vi "6733_write_waveform_2014.11.21.vi"(8 "Error In":errorcluster, 9 "Control Reference \nCluster Input":T1, 11 "Red MOT 87 Inputs 2":T2={"Active Device"="6733_Red_87", "Active Channels"=[TRUE, TRUE, TRUE, TRUE, FALSE, FALSE, FALSE, FALSE], "Waveform Parameters"=[[{"Function"=enum."Exponential", "Initial"=0.0, "Final"=0.0, "Degree"=1.0, "Nickname"="", "Conversion"=enum."B Field Grad (G/cm)", "Constant"=0.0}, {"Function"=enum."Exponential", "Initial"=0.0, "Final"=0.0, "Degree"=1.0, "Nickname"="", "Conversion"=enum."B Field Grad (G/cm)", "Constant"=0.0}, {"Function"=enum."Exponential", "Initial"=0.0, "Final"=0.0, "Degree"=1.0, "Nickname"="", "Conversion"=enum."B Field Grad (G/cm)", "Constant"=0.0}, {"Function"=enum."Exponential", "Initial"=0.0, "Final"=0.0, "Degree"=1.0, "Nickname"="", "Conversion"=enum."B Field Grad (G/cm)", "Constant"=0.0}, {"Function"=enum."Exponential", "Initial"=0.0, "Final"=0.0, "Degree"=1.0, "Nickname"="", "Conversion"=enum."B Field Grad (G/cm)", "Constant"=0.0}, {"Function"=enum."Exponential", "Initial"=0.0, "Final"=0.0, "Degree"=1.0, "Nickname"="", "Conversion"=enum."B Field Grad (G/cm)", "Constant"=0.0}], [{"Function"=enum."Exponential", "Initial"=0.0, "Final"=0.0, "Degree"=1.0, "Nickname"="", "Conversion"=enum."B Field Grad (G/cm)", "Constant"=0.0}, {"Function"=enum."Exponential", "Initial"=0.0, "Final"=0.0, "Degree"=1.0, "Nickname"="", "Conversion"=enum."B Field Grad (G/cm)", "Constant"=0.0}, {"Function"=enum."Exponential", "Initial"=0.0, "Final"=0.0, "Degree"=1.0, "Nickname"="", "Conversion"=enum."B Field Grad (G/cm)", "Constant"=0.0}, {"Function"=enum."Exponential", "Initial"=0.0, "Final"=0.0, "Degree"=1.0, "Nickname"="", "Conversion"=enum."B Field Grad (G/cm)", "Constant"=0.0}, {"Function"=enum."Exponential", "Initial"=0.0, "Final"=0.0, "Degree"=1.0, "Nickname"="", "Conversion"=enum."B Field Grad (G/cm)", "Constant"=0.0}, {"Function"=enum."Exponential", "Initial"=0.0, "Final"=0.0, "Degree"=1.0, "Nickname"="", "Conversion"=enum."B Field Grad (G/cm)", "Constant"=0.0}], [{"Function"=enum."Exponential", "Initial"=0.0, "Final"=0.0, "Degree"=1.0, "Nickname"="", "Conversion"=enum."B Field Grad (G/cm)", "Constant"=0.0}, {"Function"=enum."Exponential", "Initial"=0.0, "Final"=0.0, "Degree"=1.0, "Nickname"="", "Conversion"=enum."B Field Grad (G/cm)", "Constant"=0.0}, {"Function"=enum."Exponential", "Initial"=0.0, "Final"=0.0, "Degree"=1.0, "Nickname"="", "Conversion"=enum."B Field Grad (G/cm)", "Constant"=0.0}, {"Function"=enum."Exponential", "Initial"=0.0, "Final"=0.0, "Degree"=1.0, "Nickname"="", "Conversion"=enum."B Field Grad (G/cm)", "Constant"=0.0}, {"Function"=enum."Exponential", "Initial"=0.0, "Final"=0.0, "Degree"=1.0, "Nickname"="", "Conversion"=enum."B Field Grad (G/cm)", "Constant"=0.0}, {"Function"=enum."Exponential", "Initial"=0.0, "Final"=0.0, "Degree"=1.0, "Nickname"="", "Conversion"=enum."B Field Grad (G/cm)", "Constant"=0.0}], [{"Function"=enum."Exponential", "Initial"=0.0, "Final"=0.0, "Degree"=1.0, "Nickname"="", "Conversion"=enum."B Field Grad (G/cm)", "Constant"=0.0}, {"Function"=enum."Exponential", "Initial"=0.0, "Final"=0.0, "Degree"=1.0, "Nickname"="", "Conversion"=enum."B Field Grad (G/cm)", "Constant"=0.0}, {"Function"=enum."Exponential", "Initial"=0.0, "Final"=0.0, "Degree"=1.0, "Nickname"="", "Conversion"=enum."B Field Grad (G/cm)", "Constant"=0.0}, {"Function"=enum."Exponential", "Initial"=0.0, "Final"=0.0, "Degree"=1.0, "Nickname"="", "Conversion"=enum."B Field Grad (G/cm)", "Constant"=0.0}, {"Function"=enum."Exponential", "Initial"=0.0, "Final"=0.0, "Degree"=1.0, "Nickname"="", "Conversion"=enum."B Field Grad (G/cm)", "Constant"=0.0}, {"Function"=enum."Exponential", "Initial"=0.0, "Final"=0.0, "Degree"=1.0, "Nickname"="", "Conversion"=enum."B Field Grad (G/cm)", "Constant"=0.0}], [{"Function"=enum."Exponential", "Initial"=0.0, "Final"=0.0, "Degree"=1.0, "Nickname"="", "Conversion"=enum."B Field Grad (G/cm)", "Constant"=0.0}, {"Function"=enum."Exponential", "Initial"=0.0, "Final"=0.0, "Degree"=1.0, "Nickname"="", "Conversion"=enum."B Field Grad (G/cm)", "Constant"=0.0}, {"Function"=enum."Exponential", "Initial"=0.0, "Final"=0.0, "Degree"=1.0, "Nickname"="", "Conversion"=enum."B Field Grad (G/cm)", "Constant"=0.0}, {"Function"=enum."Exponential", "Initial"=0.0, "Final"=0.0, "Degree"=1.0, "Nickname"="", "Conversion"=enum."B Field Grad (G/cm)", "Constant"=0.0}, {"Function"=enum."Exponential", "Initial"=0.0, "Final"=0.0, "Degree"=1.0, "Nickname"="", "Conversion"=enum."B Field Grad (G/cm)", "Constant"=0.0}, {"Function"=enum."Exponential", "Initial"=0.0, "Final"=0.0, "Degree"=1.0, "Nickname"="", "Conversion"=enum."B Field Grad (G/cm)", "Constant"=0.0}], [{"Function"=enum."Exponential", "Initial"=0.0, "Final"=0.0, "Degree"=1.0, "Nickname"="", "Conversion"=enum."B Field Grad (G/cm)", "Constant"=0.0}, {"Function"=enum."Exponential", "Initial"=0.0, "Final"=0.0, "Degree"=1.0, "Nickname"="", "Conversion"=enum."B Field Grad (G/cm)", "Constant"=0.0}, {"Function"=enum."Exponential", "Initial"=0.0, "Final"=0.0, "Degree"=1.0, "Nickname"="", "Conversion"=enum."B Field Grad (G/cm)", "Constant"=0.0}, {"Function"=enum."Exponential", "Initial"=0.0, "Final"=0.0, "Degree"=1.0, "Nickname"="", "Conversion"=enum."B Field Grad (G/cm)", "Constant"=0.0}, {"Function"=enum."Exponential", "Initial"=0.0, "Final"=0.0, "Degree"=1.0, "Nickname"="", "Conversion"=enum."B Field Grad (G/cm)", "Constant"=0.0}, {"Function"=enum."Exponential", "Initial"=0.0, "Final"=0.0, "Degree"=1.0, "Nickname"="", "Conversion"=enum."B Field Grad (G/cm)", "Constant"=0.0}], [{"Function"=enum."Exponential", "Initial"=0.0, "Final"=0.0, "Degree"=1.0, "Nickname"="", "Conversion"=enum."B Field Grad (G/cm)", "Constant"=0.0}, {"Function"=enum."Exponential", "Initial"=0.0, "Final"=0.0, "Degree"=1.0, "Nickname"="", "Conversion"=enum."B Field Grad (G/cm)", "Constant"=0.0}, {"Function"=enum."Exponential", "Initial"=0.0, "Final"=0.0, "Degree"=1.0, "Nickname"="", "Conversion"=enum."B Field Grad (G/cm)", "Constant"=0.0}, {"Function"=enum."Exponential", "Initial"=0.0, "Final"=0.0, "Degree"=1.0, "Nickname"="", "Conversion"=enum."B Field Grad (G/cm)", "Constant"=0.0}, {"Function"=enum."Exponential", "Initial"=0.0, "Final"=0.0, "Degree"=1.0, "Nickname"="", "Conversion"=enum."B Field Grad (G/cm)", "Constant"=0.0}, {"Function"=enum."Exponential", "Initial"=0.0, "Final"=0.0, "Degree"=1.0, "Nickname"="", "Conversion"=enum."B Field Grad (G/cm)", "Constant"=0.0}], [{"Function"=enum."Exponential", "Initial"=0.0, "Final"=0.0, "Degree"=1.0, "Nickname"="", "Conversion"=enum."B Field Grad (G/cm)", "Constant"=0.0}, {"Function"=enum."Exponential", "Initial"=0.0, "Final"=0.0, "Degree"=1.0, "Nickname"="", "Conversion"=enum."B Field Grad (G/cm)", "Constant"=0.0}, {"Function"=enum."Exponential", "Initial"=0.0, "Final"=0.0, "Degree"=1.0, "Nickname"="", "Conversion"=enum."B Field Grad (G/cm)", "Constant"=0.0}, {"Function"=enum."Exponential", "Initial"=0.0, "Final"=0.0, "Degree"=1.0, "Nickname"="", "Conversion"=enum."B Field Grad (G/cm)", "Constant"=0.0}, {"Function"=enum."Exponential", "Initial"=0.0, "Final"=0.0, "Degree"=1.0, "Nickname"="", "Conversion"=enum."B Field Grad (G/cm)", "Constant"=0.0}, {"Function"=enum."Exponential", "Initial"=0.0, "Final"=0.0, "Degree"=1.0, "Nickname"="", "Conversion"=enum."B Field Grad (G/cm)", "Constant"=0.0}]], "Active Phases"=[TRUE, TRUE, TRUE, FALSE, FALSE, FALSE], "Phase Times"=[0.1, 0.1, 0.1], "Trigger Channel"="/6733_Red_87/PFI0"} {"Phase Times" format="%.0p"; "Waveform Parameters"."Degree" min=1.0}) -> (0 "error out":errorcluster, 2 "counter task out":refnum<k21>, 3 "waveform task out":refnum<k21>)   [LabVIEW 2016]
uses:
  6733_Red_MOT/6733_control_panel.ctl
  6733_Red_MOT/6733_waveform_parameter_array.ctl
  6733_Red_MOT/6733_waveform_item.ctl
  6733_Red_MOT/Neutral_voltage_conversion_control.ctl
  Controls/6733/Trigger_Channel_Selector.ctl
  Control 1.ctl
  <vilib>/DAQmx/write.llb/DAQmx Write (Analog 1D DBL NChan 1Samp).vi
  <vilib>/DAQmx/write.llb/DAQmx Write (Analog 1D Wfm NChan NSamp).vi
  <vilib>/DAQmx/miscellaneous.llb/DAQmx Fill In Error Info.vi
  <vilib>/Waveform/WDTOps.llb/WDT Append Waveforms DBL.vi
  <vilib>/Waveform/WDTOps.llb/WDT Scale Delta t DBL.vi
  <vilib>/DAQmx/configure/timing.llb/DAQmx Timing (Sample Clock).vi
  <vilib>/DAQmx/create/channels.llb/DAQmx Create Channel (CO-Pulse Generation-Frequency).vi
  <vilib>/DAQmx/configure/timing.llb/DAQmx Timing (Implicit).vi
  <vilib>/DAQmx/configure/trigger.llb/DAQmx Start Trigger (Digital Edge).vi
  <resource>/objmgr/daqmx.rc
panel:
  out "Total Time":dbl
  out "Sample Rate":dbl
  out "Waveforms":waveform(dbl)[](array[waveform])
  out "Max Sample Rate":dbl=1000000.0
  out "Num Inactive":i32
  out "Num  Active":i32
  out "Inactive Channels":tag[](array[tag])
  out "Active Channels":tag[](array[tag])
  out "Samples Written":dbl
  out "Voltage Maximum":dbl
  out "Voltage Minimum":dbl
  out "AO.PhysicalChans":tag[](array[tag])
  out "Active Device":tag
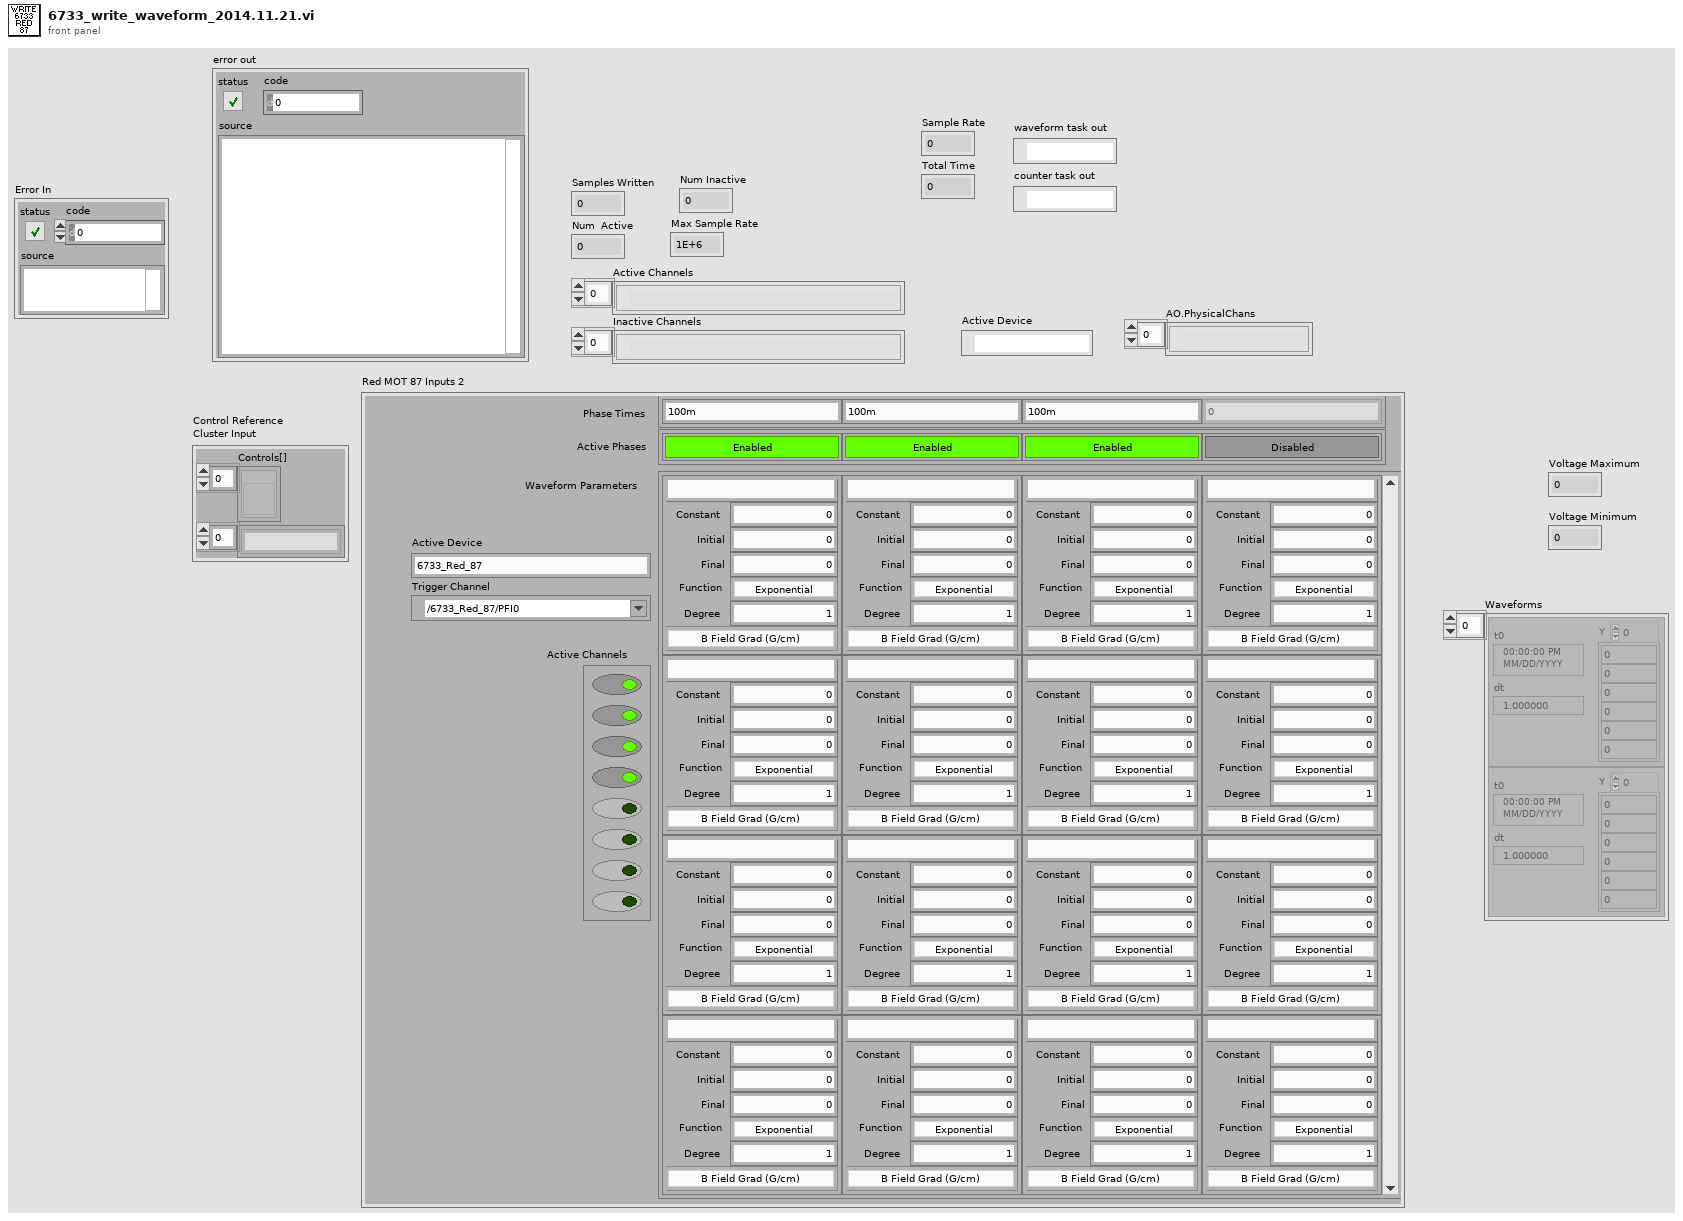
[diagram p1: front panel]
types:
  T1 = cluster{"Controls[]":refnum<vi>[], "Control Names":string[]}
  T2 = typedef "6733_control_panel.ctl" = cluster{"Active Device":string, "Active Channels":bool[], "Waveform Parameters":T3, "Active Phases":bool[], "Phase Times":dbl[], "Trigger Channel":T6}
  T3 = typedef "6733_waveform_parameter_array.ctl" = T4[][]
  T4 = typedef "6733_waveform_item.ctl" = cluster{"Function":enum16{"Polynomial", "Exponential", "Constant", "Tanh"}, "Initial":dbl, "Final":dbl, "Degree":dbl, "Nickname":string, "Conversion":T5, "Constant":dbl}
  T5 = typedef "Neutral_voltage_conversion_control.ctl" = enum16{"Volts", "B Field Grad (G/cm)", "Red Boson Cntr Freq (MHz)", "Red Boson Dither Amp (kHz)", "Red Boson Power (mW)", "Red 87 Trap Cntr Freq (MHz)", "Red 87 Trap Dither Amp (kHz)", "Red 87 Trap Power (mW)", "Red 87 Stir Cntr Freq (MHz)", "Red 87 Stir Dither Amp (kHz)", "Red 87 Stir Power (mW)", "ODT Sheet Trap Power (W)", "ODT Loading Trap Power (W)"}
  T6 = typedef "Trigger_Channel_Selector.ctl" = tag
  T7 = typedef "Control 1.ctl" = enum16{"Initialize", "Get Device Information", "Get Active/Inactive Channels", "Maximize Samples / Channel", "Calculate Waveforms", "Check for Problems", "Update Front Panel", "Clear Old Tasks", "Write Initialization to Cards", "Write Waveform to Cards"}
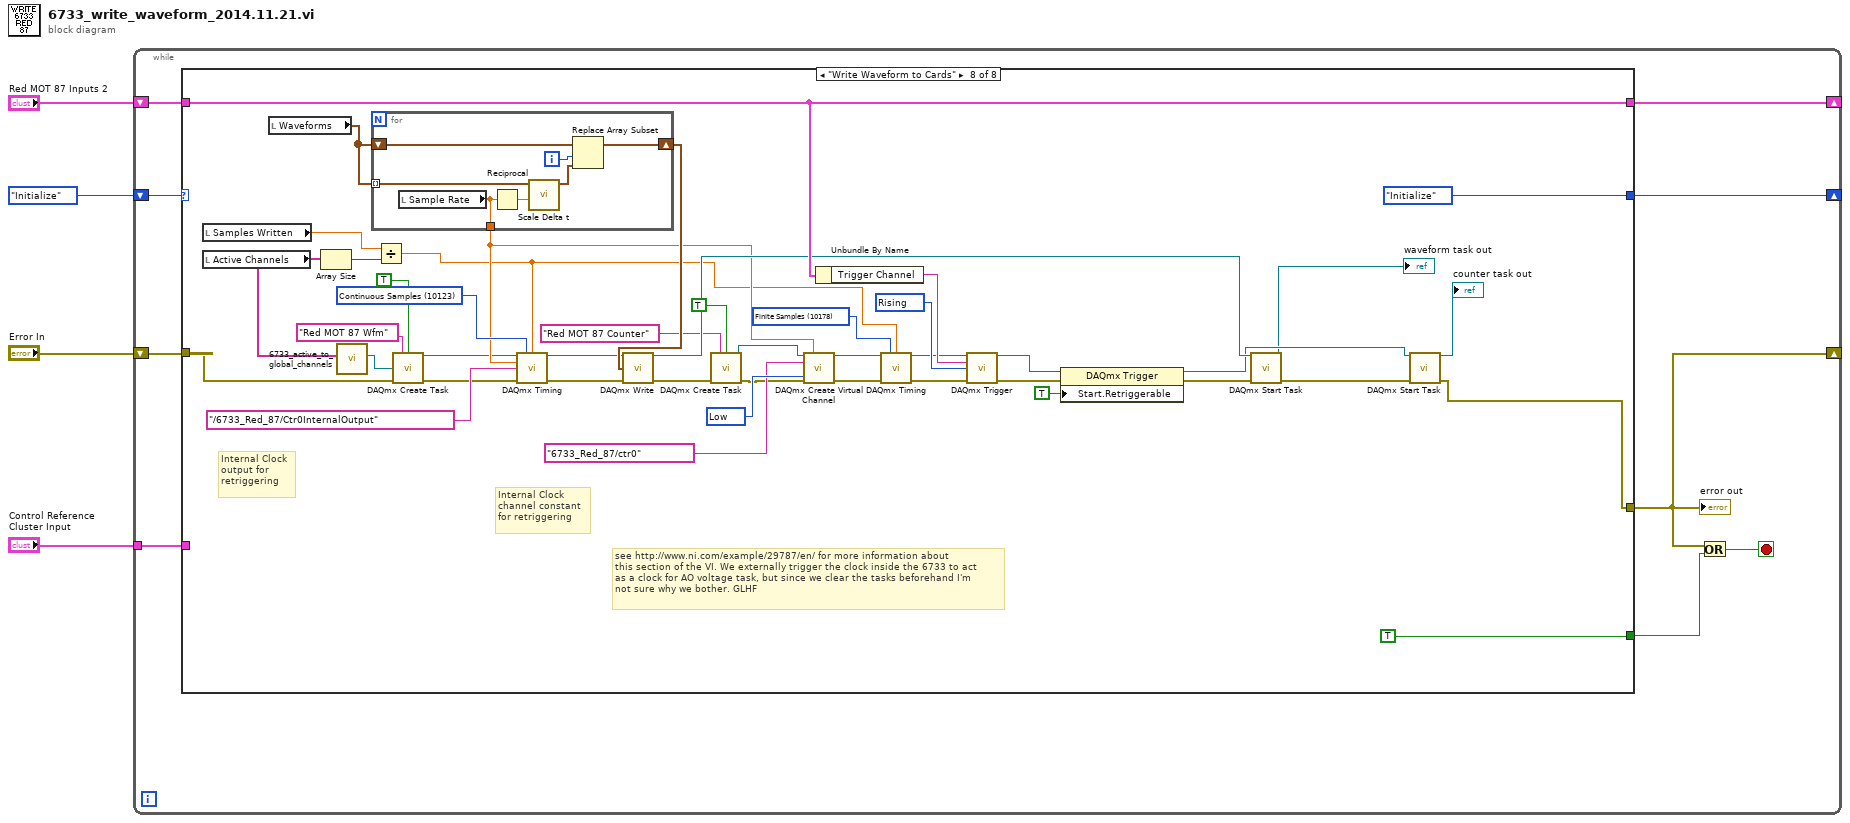
[diagram p0: block diagram]
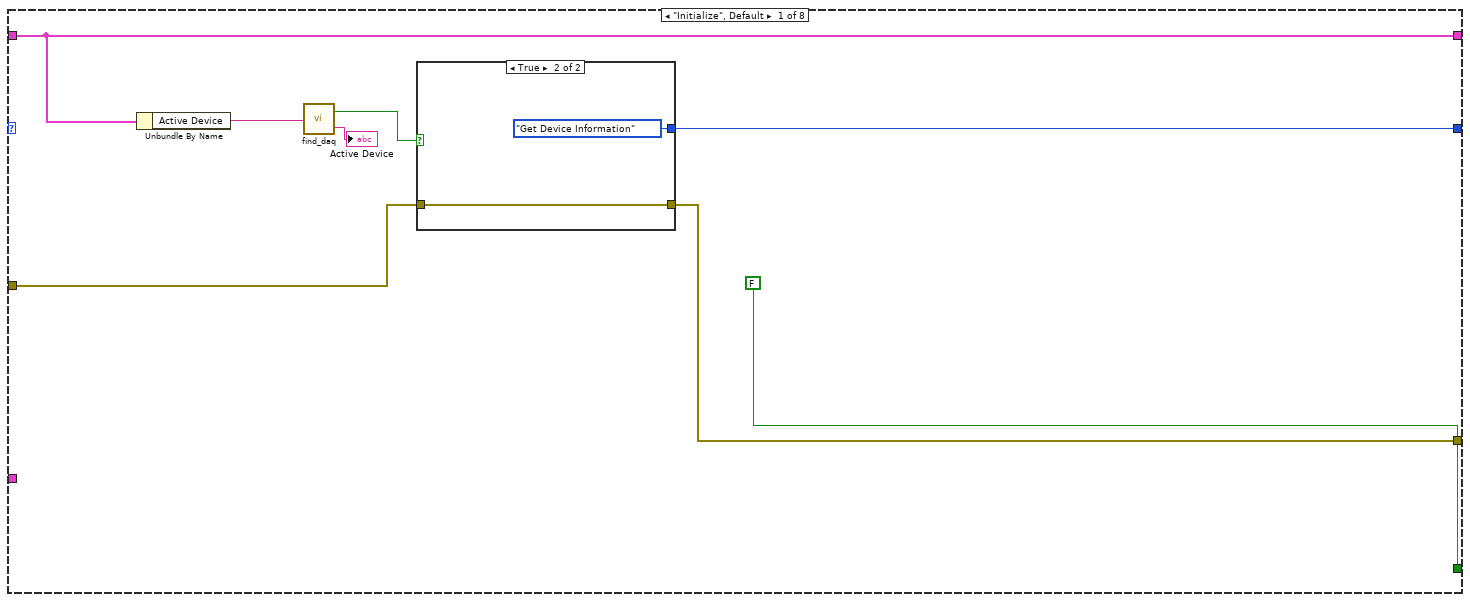
[diagram p2: hidden frame]
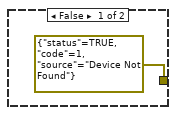
[diagram p3: hidden frame]
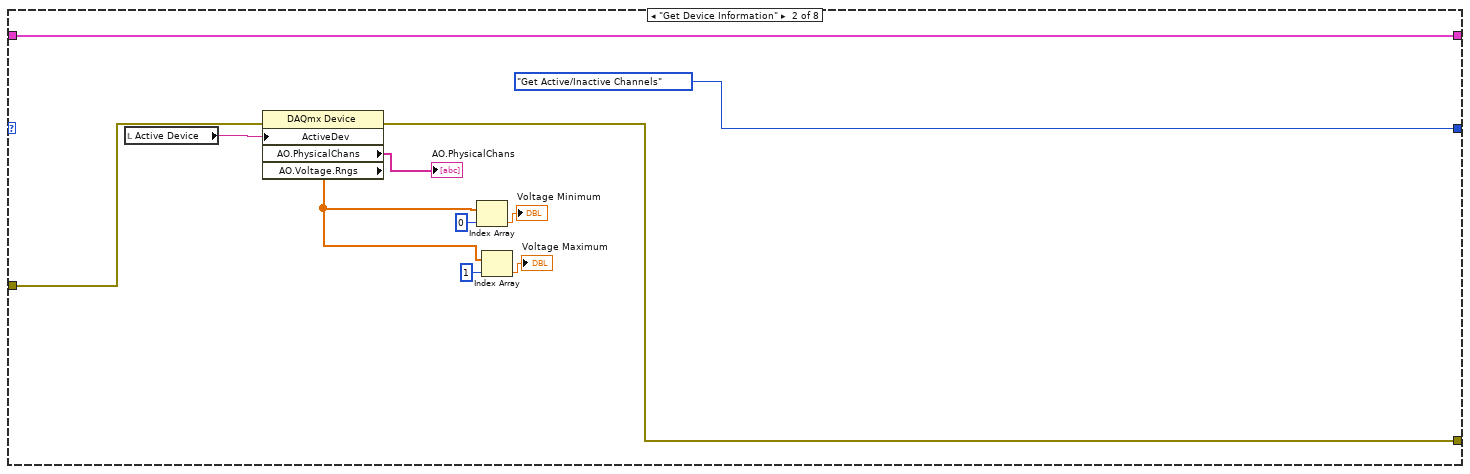
[diagram p4: hidden frame]
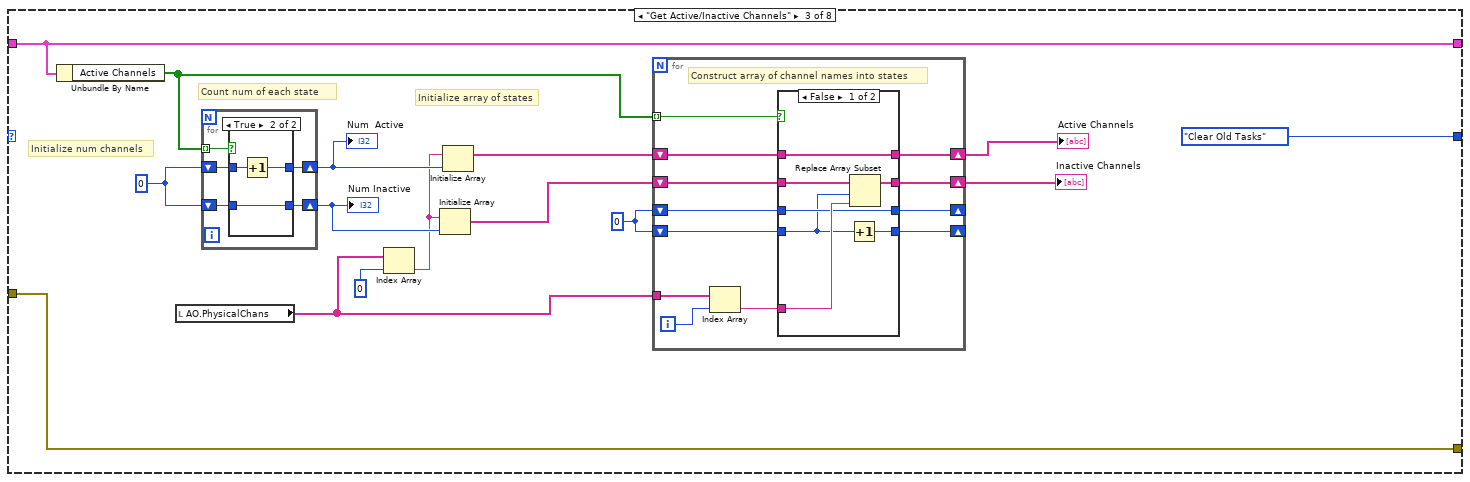
[diagram p5: hidden frame]
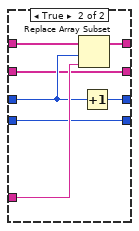
[diagram p6: hidden frame]
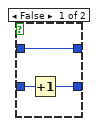
[diagram p7: hidden frame]
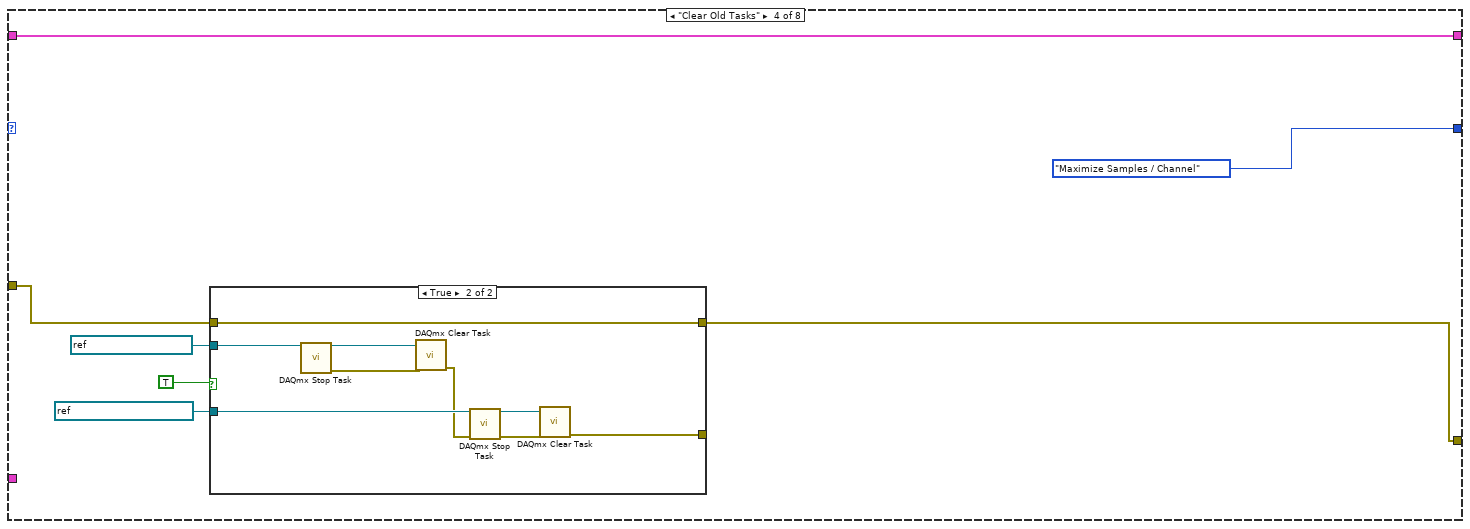
[diagram p8: hidden frame]
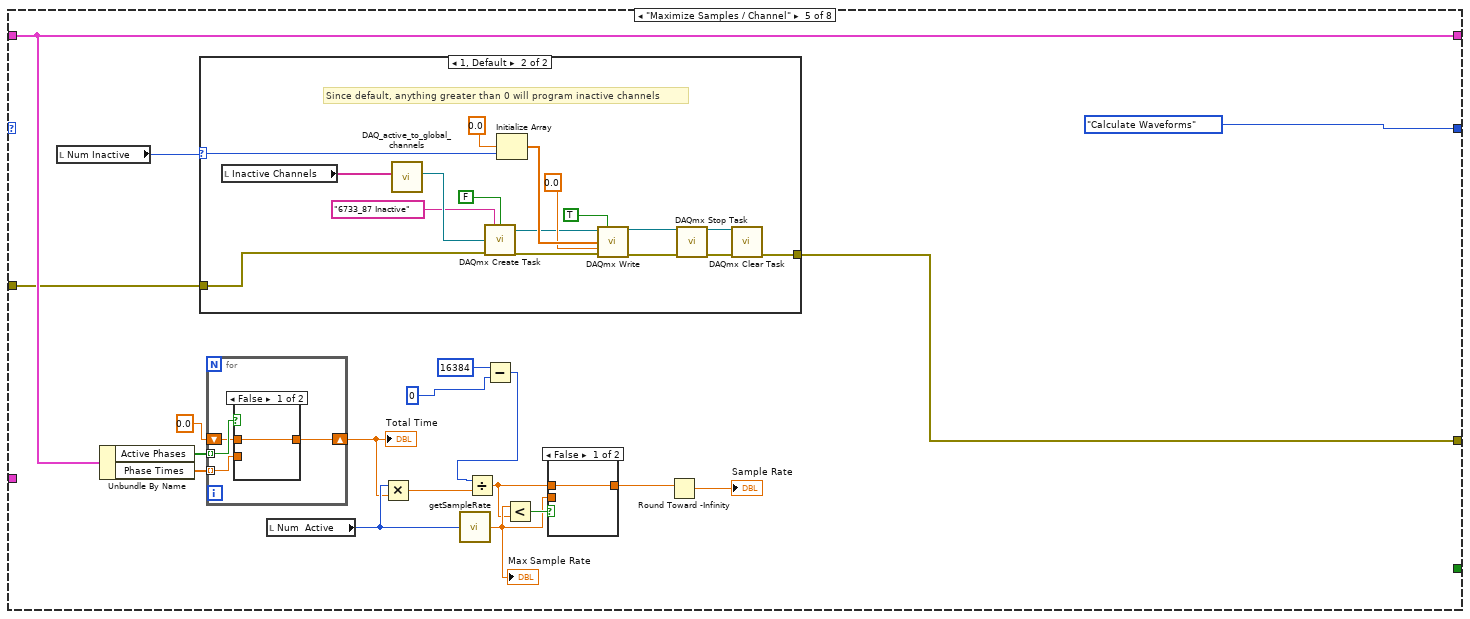
[diagram p10: hidden frame]
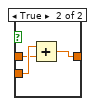
[diagram p13: hidden frame]
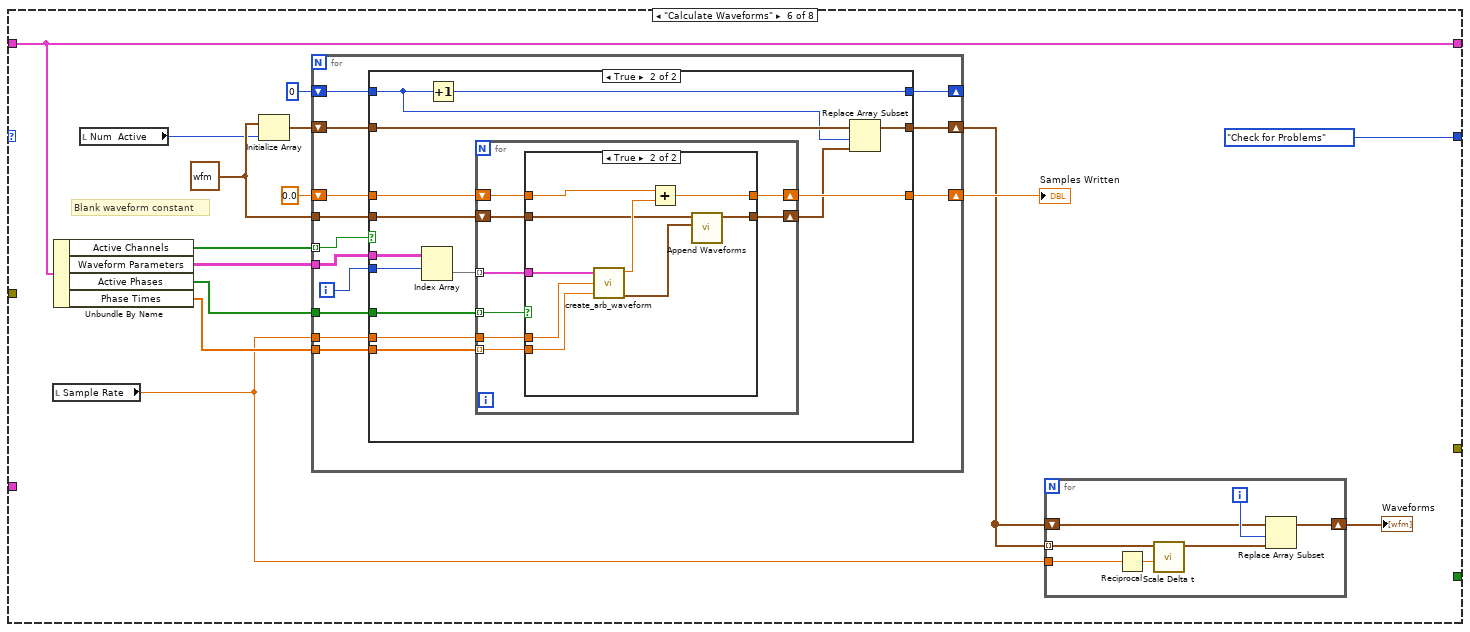
[diagram p14: hidden frame]
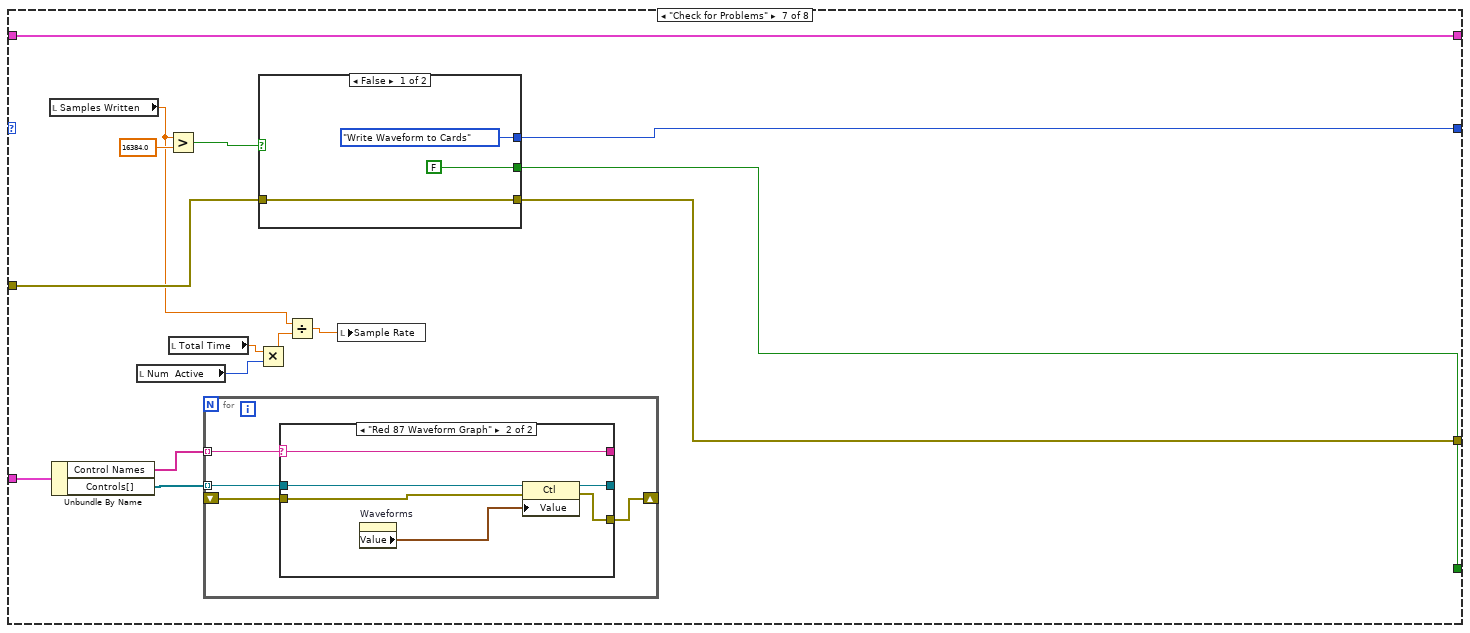
[diagram p17: hidden frame]
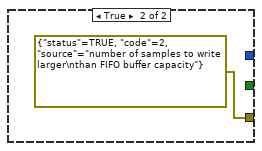
[diagram p19: hidden frame]
diagram:
  n1 = while {
    shift-right: [w5] -> _
    shift-left: "Error In" -> [w11]
    shift-right: [w10] -> _
    shift-left: Control_1."Initialize" -> [w13]
    shift-right: [w8] -> _
    shift-left: "Red MOT 87 Inputs 2" -> [w12]
    tunnel: "Control Reference \nCluster Input" -> [w6]
    stop <- w9 stop-if-true
    n2 = case shown="\"Write Waveform to Cards\"" w13 {
      tunnel: w12 -> [w15 w35 w41 w90 w121 w163 w233 w296]
      tunnel: [w18 w26 w50 w93 w123 _ w234 w273] -> w5
      tunnel: w11 -> [w17 w34 w50 w92 w106 _ w235 w270]
      tunnel: [w16 Control_1."Get Active/Inactive Channels" Control_1."Clear Old Tasks" Control_1."Maximize Samples / Channel" Control_1."Calculate Waveforms" Control_1."Check for Problems" w232 Control_1."Initialize"] -> w10
      tunnel: [w15 w35 w41 w90 w121 w163 w233 w296] -> w8
      tunnel: [FALSE ("y") _ _ _ _ _ w231 TRUE ("y")] -> w7
      tunnel: w6 -> [_ _ _ _ _ _ w223 _]
      frame "Initialize", Default {
        n3 = Unbundle By Name(w15) -> ("Active Device"=w21:string)
        n4 = call "find_daq.vi"("Device Name"=w21) -> ("Device Present"=w19:bool, "DAQmx Device Name"=→"Active Device":tag)
        n5 = case shown="True" w19 {
          tunnel: [errorcluster {"status"=TRUE, "code"=1, "source"="Device Not Found"} ("error in (no error)") w24] -> w18
          tunnel: w17 -> [_ w24]
          tunnel: [_ Control_1."Get Device Information"] -> w16
          frame False {
          }
          frame True {
          }
        }
      }
      frame "Get Device Information" {
        n6 = local read "Active Device"() -> (w33:tag)
        n7 = property class="DAQmx Device"(error in=w34, "ActiveDev"=w33) -> (error out=w26:errorcluster, "AO.PhysicalChans"=→"AO.PhysicalChans":tag[], "AO.Voltage.Rngs"=w28:dbl[])  [unwired: 1 in, 1 out]
        n8 = Index Array(array=w28, index=0) -> (element=→"Voltage Minimum":dbl)
        n9 = Index Array(array=w28, index=1) -> (element=→"Voltage Maximum":dbl)
      }
      frame "Get Active/Inactive Channels" {
        w37 = 0 ("index")
        w36 = 0
        # "Initialize array of states"
        # "Count num of each state"
        # "Initialize num channels"
        n10 = Unbundle By Name(w41) -> ("Active Channels"=w49:bool[])
        n11 = local read "AO.PhysicalChans"() -> (w43:tag[])
        n12 = for {
          shift-right: [w81] -> w48
          shift-left: w36 -> [w80]
          shift-right: [w79] -> w47
          shift-left: w36 -> [w78]
          tunnel: w49 -> [w77] mode=indexing
          n13 = case shown="True" w77 {
            tunnel: [w82 w87] -> w81
            tunnel: w80 -> [w82 w86]
            tunnel: [w84 w85] -> w79
            tunnel: w78 -> [w83 w85]
            frame False {
              n14 = Increment(x=w83) -> (x+1=w84:i32)
            }
            frame True {
              n15 = Increment(x=w86) -> (x+1=w87:i32)
            }
          }
        }
        "Num  Active" <- w48
        "Num Inactive" <- w47
        n16 = Index Array(array=w43, index=0) -> (element=w44:tag)
        n17 = Initialize Array(w44, w47) -> (w42:tag[])
        n18 = Initialize Array(w44, w48) -> (w46:tag[])
        n19 = for {
          tunnel: w49 -> [w62] mode=indexing
          shift-right: [w59] -> w40
          shift-left: w46 -> [w60]
          tunnel: w43 -> [w57]
          shift-right: [w55] -> w39
          shift-left: w42 -> [w56]
          shift-right: [w53] -> _
          shift-left: w37 -> [w54]
          shift-right: [w51] -> _
          shift-left: w37 -> [w52]
          i -> [w61]
          # "Construct array of channel names into states"
          n20 = Index Array(array=w57, index=w61) -> (element=w58:tag)
          n21 = case shown="False" w62 {
            tunnel: w60 -> [w63 w76]
            tunnel: [w63 w75] -> w59
            tunnel: w58 -> [w69 w74]
            tunnel: w56 -> [w68 w70]
            tunnel: [w67 w70] -> w55
            tunnel: w54 -> [w66 w73]
            tunnel: [w66 w72] -> w53
            tunnel: w52 -> [w65 w71]
            tunnel: [w64 w71] -> w51
            frame False {
              n22 = Increment(x=w65) -> (x+1=w64:i32)
              n23 = Replace Array Subset(array=w68, new element=w69, index=w65) -> (w67:tag[])
            }
            frame True {
              n24 = Replace Array Subset(array=w76, new element=w74, index=w73) -> (w75:tag[])
              n25 = Increment(x=w73) -> (x+1=w72:i32)
            }
          }
        }
        "Active Channels" <- w40
        "Inactive Channels" <- w39
      }
      frame "Clear Old Tasks" {
        n26 = case shown="True" TRUE {
          tunnel: refnum<k21> "Red MOT 87 Wfm" ("Waveform Task In") -> [_ w104]
          tunnel: refnum<k21> "Red MOT 87 Counter" ("Control Task In") -> [_ w102]
          tunnel: [w95 w100] -> w93
          tunnel: w92 -> [w95 w100]
          tunnel: [_ w96] -> _
          frame False {
          }
          frame True {
            n27 = call <vilib>:"DAQmx Stop Task.vi"("task/channels in"=w104) -> ("task out"=w103:refnum<k21>, "error out"=w99:errorcluster)  [unwired: 13 in]
            n28 = call <vilib>:"DAQmx Clear Task.vi"("task in"=w103, "error in"=w99) -> ("error out"=w98:errorcluster)  [unwired: 13 in]
            n29 = call <vilib>:"DAQmx Stop Task.vi"("task/channels in"=w102, "error in"=w98) -> ("task out"=w101:refnum<k21>, "error out"=w97:errorcluster)  [unwired: 12 in]
            n30 = call <vilib>:"DAQmx Clear Task.vi"("task in"=w101, "error in"=w97) -> ("error out"=w96:errorcluster)  [unwired: 13 in]
          }
        }
      }
      frame "Maximize Samples / Channel" {
        n31 = local read "Num Inactive"() -> (w105:i32)
        n32 = Unbundle By Name(w121) -> ("Active Phases"=w120:bool[], "Phase Times"=w119:dbl[])
        n33 = case shown="1, Default" w105 {
          selector: w105 -> [_ w125]
          tunnel: [w124 w137] -> w123
          tunnel: w106 -> [w124 w132]
          frame 0 {
          }
          frame 1, Default {
            # "Since default, anything greater than 0 will program inactive channels"
            n34 = local read "Inactive Channels"() -> (w126:tag[])
            n35 = call "DAQ_active_to_global_channels.vi"("Active Channels"=w126) -> ("Global Channels"=w131:refnum<k21>)  [unwired: 10 in]
            n36 = call <vilib>:"DAQmx Create Task.vi"("new task name"="6733_87 Inactive", "auto cleanup"=FALSE, "global virtual channels"=w131, "error in"=w132) -> ("task out"=w127:refnum<k21>, "error out"=w130:errorcluster)  [unwired: 10 in]
            n37 = Initialize Array(0.0 ("element"), w125) -> (w140:dbl[])
            n38 = call-poly <vilib>:"DAQmx Write.vi"("task/channels in"=w127, "auto start"=TRUE, "data"=w140, "timeout"=0.0, "error in"=w130) -> ("task out"=w135:refnum<k21>, "error out"=w136:errorcluster)  [unwired: 8 in, 1 out]
            n39 = call <vilib>:"DAQmx Stop Task.vi"("task/channels in"=w135, "error in"=w136) -> ("task out"=w139:refnum<k21>, "error out"=w138:errorcluster)  [unwired: 12 in]
            n40 = call <vilib>:"DAQmx Clear Task.vi"("task in"=w139, "error in"=w138) -> ("error out"=w137:errorcluster)  [unwired: 13 in]
          }
        }
        n41 = for {
          tunnel: w120 -> [w147] mode=indexing
          tunnel: w119 -> [w146] mode=indexing
          shift-right: [w144] -> w112
          shift-left: 0.0 -> [w145]
          n42 = case shown="False" w147 {
            tunnel: w146 -> [_ w151]
            tunnel: w145 -> [w148 w150]
            tunnel: [w148 w149] -> w144
            frame False {
            }
            frame True {
              n43 = Add(x=w151, y=w150) -> (x+y=w149:dbl)
            }
          }
        }
        "Total Time" <- w112
        n44 = local read "Num  Active"() -> (w113:i32)
        n45 = Multiply(x=w113, y=w112) -> (x*y=w114:dbl)
        n46 = call "getSampleRate.vi"("Number of active channels"=w113) -> ("Sample Rate"=w116:dbl)
        "Max Sample Rate" <- w116
        n47 = Subtract(x=16384, y=0) -> (x-y=w110:i32)
        n48 = Divide(x=w110, y=w114) -> (x/y=w115:dbl)
        n49 = Less?(x=w116, y=w115) -> (x < y?=w117:bool)
        n50 = case shown="False" w117 {
          tunnel: [w142 w143] -> w108
          tunnel: w116 -> [_ w143]
          tunnel: w115 -> [w142 _]
          frame False {
          }
          frame True {
          }
        }
        n51 = Round Toward -Infinity(1:w108) -> (0:→"Sample Rate":dbl)
      }
      frame "Calculate Waveforms" {
        w160 = waveform(dbl) {"t0"=timestamp(0 s since 1904-01-01), "dt"=1.0, "Y"=[]}
        # "Blank waveform constant"
        n52 = local read "Sample Rate"() -> (w153:dbl)
        n53 = Unbundle By Name(w163) -> ("Active Channels"=w156:bool[], "Waveform Parameters"=w166:T3, "Active Phases"=w161:bool[], "Phase Times"=w157:dbl[])
        n54 = local read "Num  Active"() -> (w155:i32)
        n55 = Initialize Array(w160, w155) -> (w158:waveform(dbl)[])
        n56 = for {
          tunnel: w156 -> [w186] mode=indexing
          tunnel: w166 -> [w184]
          shift-right: [w183] -> w165
          shift-left: 0.0 -> [w182]
          tunnel: w161 -> [w181]
          tunnel: w160 -> [w180]
          shift-right: [w178] -> _
          shift-left: 0 -> [w179]
          shift-right: [w176] -> w154
          shift-left: w158 -> [w177]
          tunnel: w157 -> [w175]
          tunnel: w153 -> [w174]
          i -> [w185]
          n57 = case shown="True" w186 {
            tunnel: w185 -> [_ w203]
            tunnel: w184 -> [_ w202]
            tunnel: [w189 w201] -> w183
            tunnel: w182 -> [w189 w200]
            tunnel: w181 -> [_ w198]
            tunnel: w180 -> [_ w197]
            tunnel: w179 -> [w188 w194]
            tunnel: [w188 w196] -> w178
            tunnel: w177 -> [w187 w195]
            tunnel: [w187 w192] -> w176
            tunnel: w175 -> [_ w191]
            tunnel: w174 -> [_ w190]
            frame False {
            }
            frame True {
              n58 = Index Array(array=w202, index (row)=w203) -> (element=w199:T4[])  [unwired: 1 in]
              n59 = Increment(x=w194) -> (x+1=w196:i32)
              n60 = for {
                shift-right: [w211] -> w201
                shift-left: w200 -> [w210]
                tunnel: w199 -> [w209] mode=indexing
                shift-right: [w207] -> w193
                shift-left: w197 -> [w208]
                tunnel: w198 -> [w206] mode=indexing
                tunnel: w191 -> [w205] mode=indexing
                tunnel: w190 -> [w204]
                n61 = case shown="True" w206 {
                  tunnel: [w213 w221] -> w211
                  tunnel: w210 -> [w213 w220]
                  tunnel: w209 -> [_ w216]
                  tunnel: w208 -> [w212 w218]
                  tunnel: [w212 w217] -> w207
                  tunnel: w205 -> [_ w215]
                  tunnel: w204 -> [_ w214]
                  frame False {
                  }
                  frame True {
                    n62 = call "create_arb_waveform.vi"("Waveform Parameters"=w216, "Sample rate"=w214, "Time"=w215) -> ("Samples to Write"=w222:dbl, "output waveform"=w219:waveform(dbl))  [unwired: 2 out]
                    n63 = Add(x=w220, y=w222) -> (x+y=w221:dbl)
                    n64 = call-poly <vilib>:"Append Waveforms.vi"("waveform B"=w219, "waveform A"=w218) -> ("waveform out"=w217:waveform(dbl))  [unwired: 8 in, 1 out]
                  }
                }
              }
              n65 = Replace Array Subset(array=w195, new element=w193, index=w194) -> (w192:waveform(dbl)[])
            }
          }
        }
        "Samples Written" <- w165
        n66 = for {
          tunnel: w154 -> [w173] mode=indexing
          shift-right: [w167] -> w152
          shift-left: w154 -> [w169]
          tunnel: w153 -> [w168]
          i -> [w171]
          n67 = Reciprocal(x=w168) -> (1/x=w172:dbl)
          n68 = call-poly <vilib>:"Scale Delta t.vi"("scale factor"=w172, "waveform in"=w173) -> ("waveform out"=w170:waveform(dbl))  [unwired: 8 in, 1 out]
          n69 = Replace Array Subset(array=w169, new element=w170, index=w171) -> (w167:waveform(dbl)[])
        }
        "Waveforms" <- w152
      }
      frame "Check for Problems" {
        n70 = local read "Samples Written"() -> (w230:dbl)
        n71 = Unbundle By Name(w223) -> ("Control Names"=w224:string[], "Controls[]"=w225:refnum<vi>[])
        n72 = local read "Num  Active"() -> (w227:i32)
        n73 = Greater?(x=w230, y=16384.0) -> (0:w237:bool)
        n74 = local read "Total Time"() -> (w228:dbl)
        n75 = for {
          tunnel: w224 -> [w241] mode=indexing
          shift-right: [w238] -> _
          shift-left: _ -> [w239]
          tunnel: w225 -> [w240] mode=indexing
          n76 = case shown="\"Red 87 Waveform Graph\"" w241 {
            selector: w241 -> [w244 w250]
            tunnel: w240 -> [w243 w247]
            tunnel: [w244 w250] -> _
            tunnel: [w243 w246] -> _
            tunnel: w239 -> [w242 w249]
            tunnel: [w242 w248] -> w238
            frame "False", Default {
            }
            frame "Red 87 Waveform Graph" {
              n77 = property on="Waveforms" class="Arr (strict)"() -> ("Value"=w245:waveform(dbl)[])  [unwired: 2 in, 2 out]
              n78 = property class="Ctl"(reference=w247, error in=w249, "Value"=w245) -> (reference out=w246:refnum<vi>, error out=w248:errorcluster)
            }
          }
        }
        n79 = Multiply(x=w228, y=w227) -> (x*y=w226:dbl)
        n80 = case shown="False" w237 {
          tunnel: w235 -> [w253 _]
          tunnel: [w253 errorcluster {"status"=TRUE, "code"=2, "source"="number of samples to write larger\nthan FIFO buffer capacity"} ("error in (no error)")] -> w234
          tunnel: [Control_1."Write Waveform to Cards" _] -> w232
          tunnel: [FALSE ("y") _] -> w231
          frame False {
          }
          frame True {
          }
        }
        n81 = Divide(x=w230, y=w226) -> (x/y=w229:dbl)
        n82 = local write "Sample Rate"(w229) -> ()
      }
      frame "Write Waveform to Cards" {
        w286 = 10280 items=["Rising"=10280, "Falling"=10171] ("edge")
        w291 = 10123 items=["Finite Samples"=10178, "Continuous Samples"=10123, "Hardware Timed Single Point"=12522] ("sample mode")
        w292 = 10178 items=["Finite Samples"=10178, "Continuous Samples"=10123, "Hardware Timed Single Point"=12522] ("sample mode")
        w295 = 10214 items=["High"=10192, "Low"=10214] ("idle state")
        # "see http://www.ni.com/example/29787/en/ for more information about\nthis section of the VI. We externally trigger the clock inside the 6733 to act\nas a clock for AO voltage task, but since we clear the tasks beforehand I'm\nnot sure why we bother. GLHF"
        # "Internal Clock\noutput for\nretriggering"
        # "Internal Clock\nchannel constant\nfor retriggering"
        n83 = local read "Samples Written"() -> (w255:dbl)
        n84 = local read "Active Channels"() -> (w258:tag[])
        n85 = local read "Waveforms"() -> (w297:waveform(dbl)[])
        n86 = Array Size(array=w258) -> (size(s)=w256:i32)
        n87 = call "6733_active_to_global_channels.vi"("Active Channels"=w258) -> ("Global Channels"=w268:refnum<k21>)  [unwired: 10 in]
        n88 = for {
          tunnel: w297 -> [w305] mode=indexing
          shift-right: [w299] -> w289
          shift-left: w297 -> [w301]
          tunnel: [w300] -> w276
          i -> [w303]
          n89 = local read "Sample Rate"() -> (w300:dbl)
          n90 = Reciprocal(x=w300) -> (1/x=w304:dbl)
          n91 = call-poly <vilib>:"Scale Delta t.vi"("scale factor"=w304, "waveform in"=w305) -> ("waveform out"=w302:waveform(dbl))  [unwired: 8 in, 1 out]
          n92 = Replace Array Subset(array=w301, new element=w302, index=w303) -> (w299:waveform(dbl)[])
        }
        n93 = Divide(x=w255, y=w256) -> (x/y=w257:dbl)
        n94 = call <vilib>:"DAQmx Create Task.vi"("new task name"="Red MOT 87 Wfm", "auto cleanup"=TRUE, "global virtual channels"=w268, "error in"=w270) -> ("task out"=w266:refnum<k21>, "error out"=w269:errorcluster)  [unwired: 10 in]
        n95 = call-poly <vilib>:"DAQmx Timing.vi"("task/channels in"=w266, "sample mode"=w291, "samples per channel"=w257, "rate"=w276, "source"=tag "/6733_Red_87/Ctr0InternalOutput", "error in"=w269) -> ("task out"=w288:refnum<k21>, "error out"=w290:errorcluster)  [unwired: 8 in]
        n96 = call-poly <vilib>:"DAQmx Write.vi"("task/channels in"=w288, "data"=w289, "error in"=w290) -> ("task out"=w280:refnum<k21>, "error out"=w265:errorcluster)  [unwired: 10 in, 1 out]
        n97 = call <vilib>:"DAQmx Create Task.vi"("new task name"="Red MOT 87 Counter", "auto cleanup"=TRUE, "error in"=w265) -> ("task out"=w260:refnum<k21>, "error out"=w264:errorcluster)  [unwired: 11 in]
        n98 = call-poly <vilib>:"DAQmx Create Virtual Channel.vi"("task in"=w260, "frequency"=w276, "counter"=tag "6733_Red_87/ctr0", "error in"=w264, "idle state"=w295) -> ("task out"=w294:refnum<k21>, "error out"=w293:errorcluster)  [unwired: 9 in]
        n99 = Unbundle By Name(w296) -> ("Trigger Channel"=w285:T6)
        n100 = call-poly <vilib>:"DAQmx Timing.vi"("task/channels in"=w294, "sample mode"=w292, "samples per channel"=w257, "error in"=w293) -> ("task out"=w284:refnum<k21>, "error out"=w287:errorcluster)  [unwired: 10 in]
        n101 = call-poly <vilib>:"DAQmx Trigger.vi"("task/channels in"=w284, "source"=w285, "edge"=w286, "error in"=w287) -> ("task out"=w282:refnum<k21>, "error out"=w283:errorcluster)  [unwired: 10 in]
        n102 = property class="DAQmx Trigger"(reference=w282, error in=w283, "Start.Retriggerable"=TRUE) -> (reference out=w277:refnum<k21>, error out=w279:errorcluster)
        n103 = call <vilib>:"DAQmx Start Task.vi"("task/channels in"=w280, "error in"=w279) -> ("task out"=→"waveform task out":refnum<k21>, "error out"=w278:errorcluster)  [unwired: 12 in]
        n104 = call <vilib>:"DAQmx Start Task.vi"("task/channels in"=w277, "error in"=w278) -> ("task out"=→"counter task out":refnum<k21>, "error out"=w273:errorcluster)  [unwired: 12 in]
      }
    }
    "error out" <- w5
    n105 = Or(x=w5, y=w7) -> (x .or. y?=w9:bool)
  }
